vi "Manipulator Control.vi"() -> ()   [LabVIEW 2018]
uses:
  <vilib>/Platform/TimedLoop/XDataNode/timing_clust.ctl
  <vilib>/Platform/TimedLoop/XDataNode/nitl_modes.ctl
  <vilib>/Platform/TimedLoop/XDataNode/wakeup.ctl
  <vilib>/Analysis/baseanly.llb/Mean (DBL).vi
  <extravilib>/ChannelInstances/Tag-a[.](dbl)/Read With Abort.vi
  <extravilib>/ChannelInstances/Tag-bool/Read With Abort.vi
  <extravilib>/ChannelInstances/Tag-a[.](dbl)/Write With Abort.vi
  <extravilib>/ChannelInstances/Tag-bool/Write With Abort.vi
  <extravilib>/ChannelInstances/Tag-a[.](dbl)/Instantiate.vi
  <extravilib>/ChannelInstances/Tag-bool/Instantiate.vi
  <extravilib>/ChannelInstances/Tag-a[.](dbl)/EndpointRead.vi
  <extravilib>/ChannelInstances/Tag-bool/EndpointRead.vi
  <extravilib>/ChannelInstances/Tag-a[.](dbl)/Endpoint.vi
  <extravilib>/ChannelInstances/Tag-bool/Endpoint.vi
  <vilib>/Platform/TimedLoop/XDataNode/XDataNode.xnode
  <extravilib>/ChannelInstances/Tag-a[.](dbl).lvlib
  <extravilib>/ChannelInstances/Tag-bool.lvlib
  <vilib>/Platform/TimedLoop/XDataNode/XDNodeRunTimeDep.lvlib
  <vilib>/Analysis/NI_AALBase.lvlib
panel:
  in  "Derivative 1":dbl(slide)=6.0 min=0.0 max=10.0 step=0.1 scale=0.0..10.0
  in  "Integral 1":dbl(slide)=10.0 min=0.0 max=100.0 step=1.0 scale=0.0..100.0
  in  "Proportional 1":dbl(slide)=85.0 min=0.0 max=200.0 step=1.0 scale=0.0..200.0
  in  "Derivative 0":dbl(slide)=6.0 min=0.0 max=10.0 step=0.1 scale=0.0..10.0
  in  "Integral 0":dbl(slide)=10.0 min=0.0 max=100.0 step=1.0 scale=0.0..100.0
  out "Mean Task-Space \nerror (cm)":dbl=0.12500458479740745
  in  "Start Test":bool
  in  "Trajectory":enum16{"Circle", "Square"}(ring)
  in  "Stop Button":bool
  out "Calibrated":bool=TRUE
  out "Number of loops \ncompleted":i32=27
  in  "Error Threshold\n (cm)":dbl=0.3 format="%#_13g"
  in  "Proportional 0":dbl(slide)=85.0 min=0.0 max=200.0 step=1.0 scale=0.0..200.0
  out "Task-space Error":dbl(graph)=0.125479420396201
  out "Motor Voltage":T1(graph)={"element[0]"=-1.413534066833547, "element[1]"=1.33132478046187, "element[2]"=0.0, "element[3]"=0.0, "element[4]"=0.0, "element[5]"=0.0, "element[6]"=0.0, "element[7]"=0.0, "element[8]"=0.0}
  out "End-effector Trajectory":cluster{dbl[], dbl[]}[](graph)=[{[0.0, 0.0, 0.0, 0.0, 0.0, 0.0, 0.0, 0.0, 0.0, 0.0, 0.0, 0.0, 0.0, 0.0, 0.0, 0.0, 0.0, 0.0, 0.0, 0.0, 0.0, 0.0, 0.0, 0.0, 0.0, 0.0, 0.0, 0.0, 0.0, 0.0, 0.0, 0.0, 0.0, 0.0, 0.0, 0.0, 0.0, 0.0, 0.0, 0.0, 0.0, 0.0, 0.0, 0.0, 0.0, 0.0, 0.0, 0.0, 0.0, 0.0, 0.0, 0.0, 0.0, 0.0, 0.0, 0.0, 0.0, 0.0, 0.0, 0.0, 0.0, 0.0, 0.0, 0.0, 0.0, 0.0, 0.0, 0.0, 0.0, 0.0, 0.0, 0.0, 0.0, 0.0, 0.0, 0.0, 0.0, 0.0, 0.0, 0.0, 0.0, 0.0, 0.0, 0.0, 0.0, 0.0, 0.0, 0.0, 0.0, 0.0, 0.0, 0.0, 0.0, 0.0, 0.0, 0.0, 0.0, 0.0, 0.0, 0.0, 0.0, 0.0, 0.0, 0.0, 0.0, 0.0, 0.0, 0.0, 0.0, 0.0, 0.0, 0.0, 0.0, 0.0, 0.0, 0.0, 0.0, 0.0, 0.0, 0.0, 0.0, 0.0, 0.0, 0.0, 0.0, 0.0, 0.0, 0.0], [10.0, 10.0, 10.0, 10.0, 10.0, 10.0, 10.0, 10.0, 10.0, 10.0, 10.0, 10.0, 10.0, 10.0, 10.0, 10.0, 10.0, 10.0, 10.0, 10.0, 10.0, 10.0, 10.0, 10.0, 10.0, 10.0, 10.0, 10.0, 10.0, 10.0, 10.0, 10.0, 10.0, 10.0, 10.0, 10.0, 10.0, 10.0, 10.0, 10.0, 10.0, 10.0, 10.0, 10.0, 10.0, 10.0, 10.0, 10.0, 10.0, 10.0, 10.0, 10.0, 10.0, 10.0, 10.0, 10.0, 10.0, 10.0, 10.0, 10.0, 10.0, 10.0, 10.0, 10.0, 10.0, 10.0, 10.0, 10.0, 10.0, 10.0, 10.0, 10.0, 10.0, 10.0, 10.0, 10.0, 10.0, 10.0, 10.0, 10.0, 10.0, 10.0, 10.0, 10.0, 10.0, 10.0, 10.0, 10.0, 10.0, 10.0, 10.0, 10.0, 10.0, 10.0, 10.0, 10.0, 10.0, 10.0, 10.0, 10.0, 10.0, 10.0, 10.0, 10.0, 10.0, 10.0, 10.0, 10.0, 10.0, 10.0, 10.0, 10.0, 10.0, 10.0, 10.0, 10.0, 10.0, 10.0, 10.0, 10.0, 10.0, 10.0, 10.0, 10.0, 10.0, 10.0, 10.0, 10.0]}, {[0.10886586911216156, 0.10886586911216156, 0.10886586911216156, 0.10886586911216156, 0.10886586911216156, 0.10338675897126315, 0.10338675897126315, 0.10886586911216156, 0.10886586911216156, 0.10886586911216156, 0.10886586911216156, 0.10886586911216156, 0.10886586911216156, 0.10338675897126315, 0.10338675897126315, 0.12367237442525791, 0.10886586911216156, 0.10886586911216156, 0.10886586911216156, 0.10886586911216156, 0.10886586911216156, 0.10338675897126315, 0.10338675897126315, 0.10338675897126315, 0.10338675897126315, 0.10338675897126315, 0.10886586911216156, 0.12914220502365836, 0.10886586911216156, 0.10886586911216156, 0.10886586911216156, 0.10886586911216156, 0.10338675897126315, 0.10338675897126315, 0.10338675897126315, 0.12914220502365836, 0.10886586911216156, 0.12914220502365836, 0.12914220502365836, 0.10338675897126315, 0.12367237442525791, 0.12367237442525791, 0.10886586911216156, 0.10886586911216156, 0.10886586911216156, 0.10886586911216156, 0.12914220502365836, 0.12914220502365836, 0.10886586911216156, 0.10886586911216156, 0.10886586911216156, 0.10886586911216156, 0.12367237442525791, 0.12367237442525791, 0.10338675897126315, 0.12914220502365836, 0.10886586911216156, 0.12914220502365836, 0.12914220502365836, 0.10886586911216156, 0.12914220502365836, 0.12914220502365836, 0.10886586911216156, 0.10886586911216156, 0.10338675897126315, 0.10886586911216156, 0.12914220502365836, 0.12914220502365836, 0.12914220502365836, 0.12914220502365836, 0.12914220502365836, 0.10886586911216156, 0.12914220502365836, 0.12367237442525791, 0.10886586911216156, 0.12367237442525791, 0.10886586911216156, 0.12914220502365836, 0.12914220502365836, 0.12914220502365836, 0.12914220502365836, 0.10886586911216156, 0.12914220502365836, 0.12914220502365836, 0.12367237442525791, 0.10886586911216156, 0.10338675897126315, 0.12914220502365836, 0.12914220502365836, 0.12914220502365836, 0.12914220502365836, 0.12914220502365836, 0.12914220502365836, 0.10886586911216156, 0.12914220502365836, 0.10886586911216156, 0.12367237442525791, 0.12367237442525791, 0.12914220502365836, 0.12367237442525791, 0.12914220502365836, 0.12914220502365836, 0.12914220502365836, 0.12914220502365836, 0.12914220502365836, 0.12914220502365836, 0.12914220502365836, 0.12914220502365836, 0.12914220502365836, 0.12367237442525791, 0.12914220502365836, 0.12914220502365836, 0.12914220502365836, 0.12914220502365836, 0.12914220502365836, 0.12914220502365836, 0.12914220502365836, 0.12914220502365836, 0.12914220502365836, 0.12914220502365836, 0.12914220502365836, 0.12914220502365836, 0.12914220502365836, 0.12914220502365836, 0.12914220502365836, 0.12914220502365836, 0.12914220502365836, 0.12914220502365836], [9.93760362602346, 9.93760362602346, 9.93760362602346, 9.93760362602346, 9.93760362602346, 9.91519089242297, 9.91519089242297, 9.93760362602346, 9.93760362602346, 9.93760362602346, 9.93760362602346, 9.93760362602346, 9.93760362602346, 9.91519089242297, 9.91519089242297, 9.896688321217006, 9.93760362602346, 9.93760362602346, 9.93760362602346, 9.93760362602346, 9.93760362602346, 9.91519089242297, 9.91519089242297, 9.91519089242297, 9.91519089242297, 9.91519089242297, 9.93760362602346, 9.919095342569769, 9.93760362602346, 9.93760362602346, 9.93760362602346, 9.93760362602346, 9.91519089242297, 9.91519089242297, 9.91519089242297, 9.919095342569769, 9.93760362602346, 9.919095342569769, 9.919095342569769, 9.91519089242297, 9.896688321217006, 9.896688321217006, 9.93760362602346, 9.93760362602346, 9.93760362602346, 9.93760362602346, 9.919095342569769, 9.919095342569769, 9.93760362602346, 9.93760362602346, 9.93760362602346, 9.93760362602346, 9.896688321217006, 9.896688321217006, 9.91519089242297, 9.919095342569769, 9.93760362602346, 9.919095342569769, 9.919095342569769, 9.93760362602346, 9.919095342569769, 9.919095342569769, 9.93760362602346, 9.93760362602346, 9.91519089242297, 9.93760362602346, 9.919095342569769, 9.919095342569769, 9.919095342569769, 9.919095342569769, 9.919095342569769, 9.93760362602346, 9.919095342569769, 9.896688321217006, 9.93760362602346, 9.896688321217006, 9.93760362602346, 9.919095342569769, 9.919095342569769, 9.919095342569769, 9.919095342569769, 9.93760362602346, 9.919095342569769, 9.919095342569769, 9.896688321217006, 9.93760362602346, 9.91519089242297, 9.919095342569769, 9.919095342569769, 9.919095342569769, 9.919095342569769, 9.919095342569769, 9.919095342569769, 9.93760362602346, 9.919095342569769, 9.93760362602346, 9.896688321217006, 9.896688321217006, 9.919095342569769, 9.896688321217006, 9.919095342569769, 9.919095342569769, 9.919095342569769, 9.919095342569769, 9.919095342569769, 9.919095342569769, 9.919095342569769, 9.919095342569769, 9.919095342569769, 9.896688321217006, 9.919095342569769, 9.919095342569769, 9.919095342569769, 9.919095342569769, 9.919095342569769, 9.919095342569769, 9.919095342569769, 9.919095342569769, 9.919095342569769, 9.919095342569769, 9.919095342569769, 9.919095342569769, 9.919095342569769, 9.919095342569769, 9.919095342569769, 9.919095342569769, 9.919095342569769, 9.919095342569769]}]
  # "Mechatronic Systems Board"
  # "Manipulator Control"
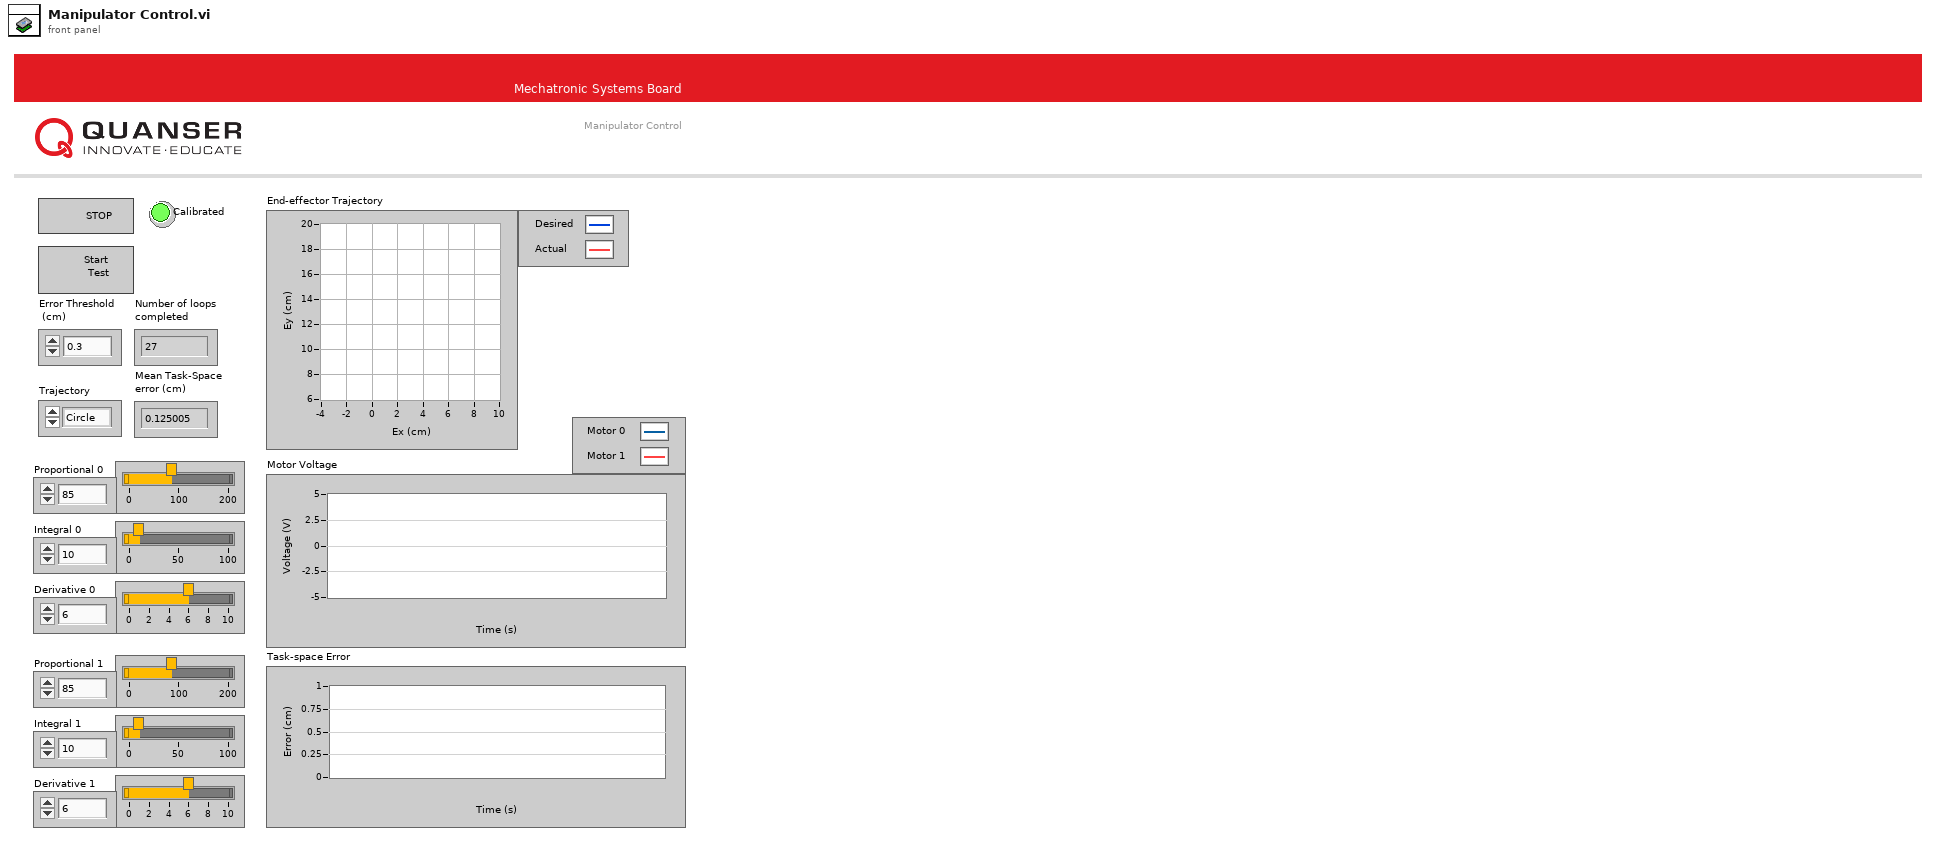
[diagram p1: front panel]
types:
  T1 = cluster{"element[0]":dbl, "element[1]":dbl, "element[2]":dbl, "element[3]":dbl, "element[4]":dbl, "element[5]":dbl, "element[6]":dbl, "element[7]":dbl, "element[8]":dbl}
  T2 = enum16{"Initialize", "Ready", "Start", "Move", "Wait", "Done"}
  T3 = typedef "QNET MS IO Cluster.ctl" = cluster{"Error":errorcluster, "Encoder Calibration Values":i32[], "Update Calibration":bool, "JPEG Resolutions":u16, "Raw Resolutions":u16, "Image Mode":enum16{"RAW RGB", "RAW Gray Scale", "JPEG"}, "FPGA Ref":refnum<k20>}
  T4 = typedef "XDNodeRunTimeDep.lvlib/timing_clust.ctl" = cluster{"Expected End [f-1]":u64, "Actual End [f-1]":u64, "Finished Late? [f-1]":bool, "Expected End [i-1]":u64, "Actual End [i-1]":u64, "Finished Late? [i-1]":bool, "Expected Start [i]":u64, "Actual Start [i]":u64, "Expected Start [f]":u64, "Actual Start [f]":u64, "Source Name":string, "Structure Name":string, "Period":i64, "Deadline":i64, "Offset":i64, "Start":i64, "Priority":i32, "Timeout":i32, "Mode":T5, "Wakeup Reason":T6, "Error":errorcluster, "Source Type":string, "Secondary Source Type":string, "Global End Time":u64, "Global Start Time":u64, "Frame Duration":u64, "Iteration Duration":u64, "Assigned CPU":i32, "I/O Scan Engine Mode":u32}
  T5 = typedef "XDNodeRunTimeDep.lvlib/nitl_modes.ctl" = enum32{"No Change", "Process missed periods, maintain original phase", "Discard missed periods, maintain original phase", "Process missed periods, ignore original phase", "Discard missed periods, ignore original phase"}
  T6 = typedef "XDNodeRunTimeDep.lvlib/wakeup.ctl" = enum32{"Normal", "Aborted", "Asynchronous wakeup", "Timing source error", "Timed loop error", "Timeout"}
  T7 = enum8{"Enabled", "Disabled", "Disabled and Grayed Out"}
  T8 = typedef "Tag-bool.lvlib/))Channel.ctl" = refnum<queue>
  T9 = typedef "Tag-a[.](dbl).lvlib/))Channel.ctl" = refnum<queue>
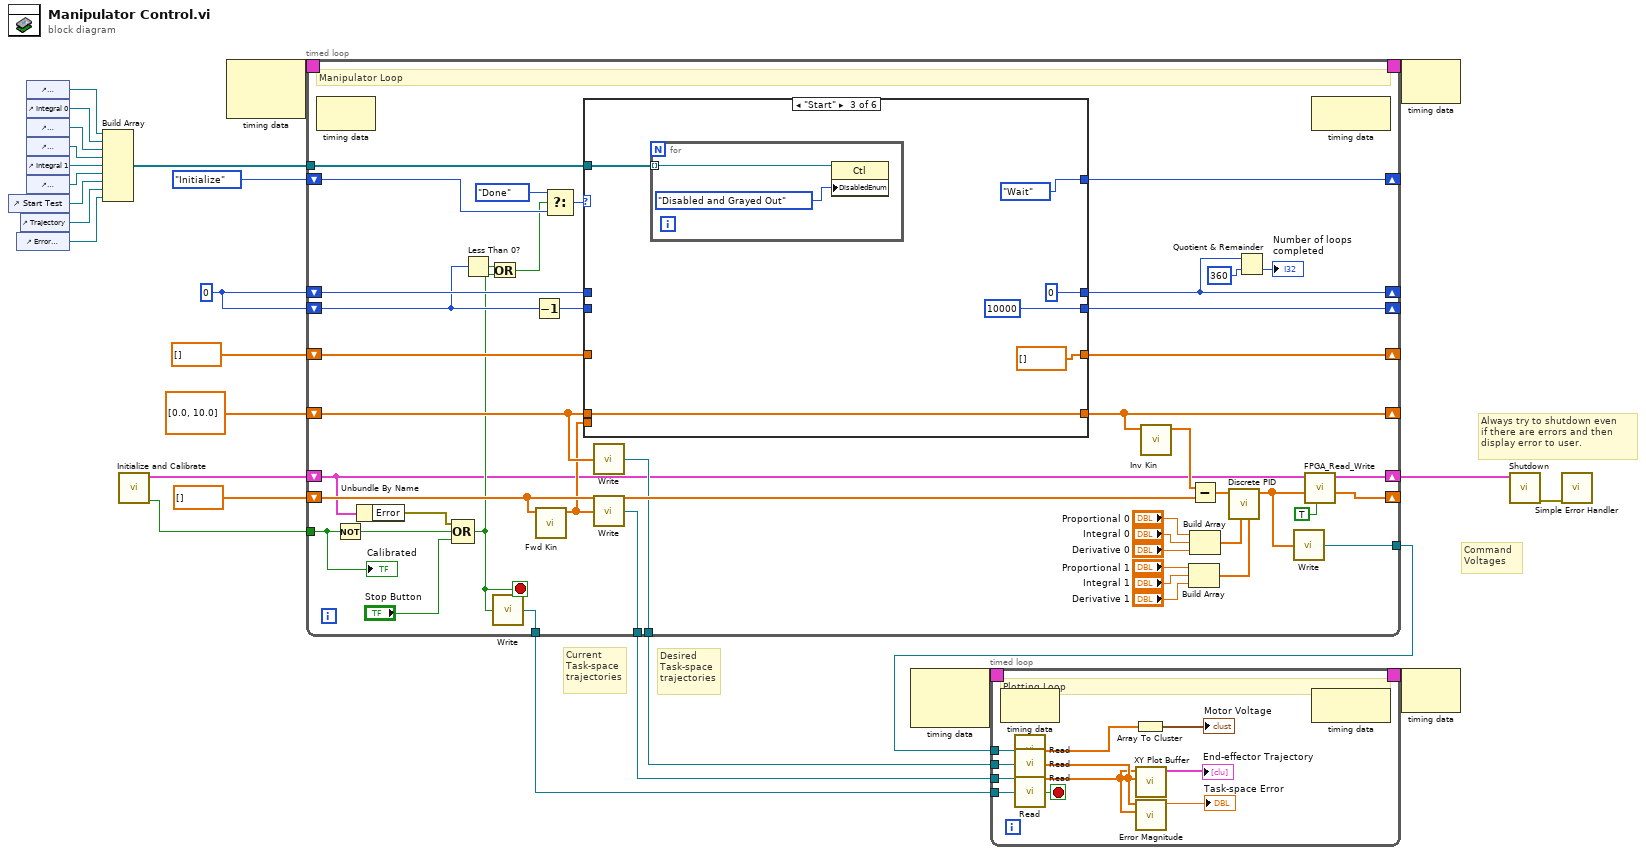
[diagram p0: block diagram]
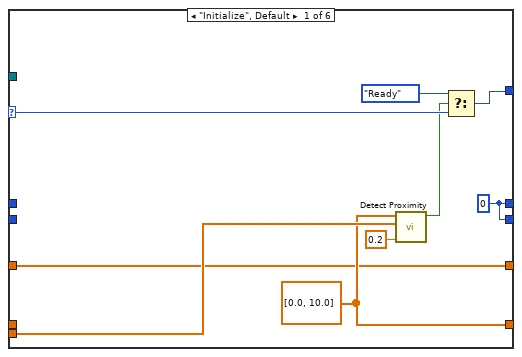
[diagram p2: hidden frame]
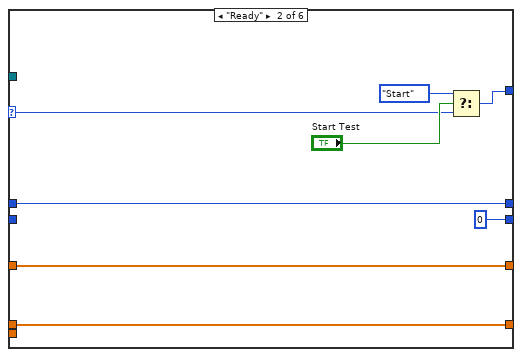
[diagram p3: hidden frame]
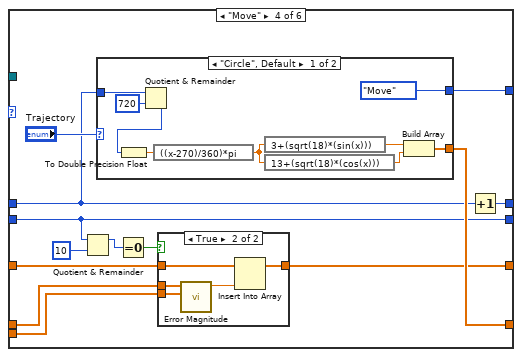
[diagram p4: hidden frame]
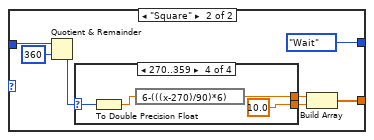
[diagram p6: hidden frame]
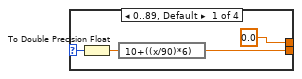
[diagram p7: hidden frame]
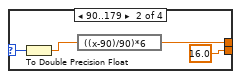
[diagram p8: hidden frame]
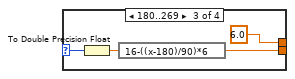
[diagram p9: hidden frame]
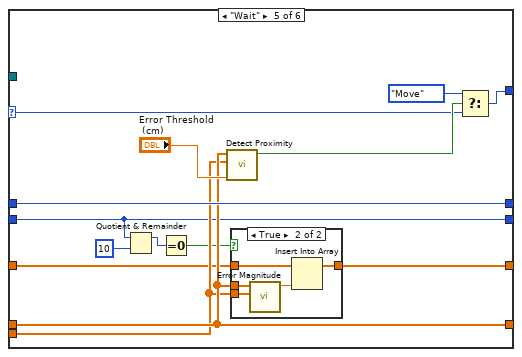
[diagram p10: hidden frame]
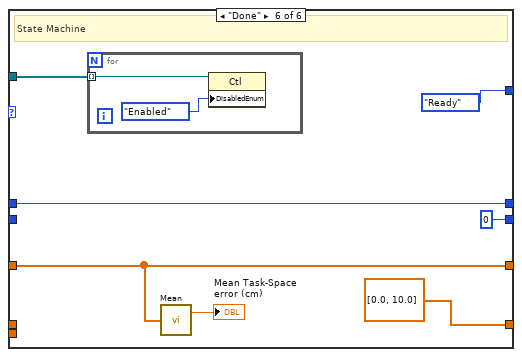
[diagram p12: hidden frame]
diagram:
  w9 = 0
  # "Command\nVoltages"
  # "Current\nTask-space\ntrajectories"
  # "Desired\nTask-space\ntrajectories"
  # "Always try to shutdown even \nif there are errors and then \ndisplay error to user."
  n1 = control-ref of="Start Test"() -> (w14:refnum<vi>)
  n2 = control-ref of="Error Threshold\n (cm)"() -> (w12:refnum<vi>)
  n3 = control-ref of="Trajectory"() -> (w13:refnum<vi>)
  n4 = control-ref of="Proportional 0"() -> (w15:refnum<vi>)
  n5 = control-ref of="Integral 0"() -> (w7:refnum<vi>)
  n6 = control-ref of="Derivative 0"() -> (w6:refnum<vi>)
  n7 = control-ref of="Proportional 1"() -> (w5:refnum<vi>)
  n8 = control-ref of="Integral 1"() -> (w4:refnum<vi>)
  n9 = control-ref of="Derivative 1"() -> (w3:refnum<vi>)
  n10 = Build Array(w15, w7, w6, w5, w4, w3, w14, w13, w12) -> (w11:refnum<vi>[])
  n11 = call "Initialize and Calibrate.vi"() -> ("Calibrated"=w19:bool, "IO Cluster"=w24:T3)  [unwired: 10 in]
  n12 = node-c288() -> (w26:T4)  [unwired: 2 in]
  n13 = timed-loop {
    timing: w26 -> [_]
    timing-out: [_] -> w25
    shift-right: [w66] -> w23
    shift-left: w24 -> [w29]
    shift-right: [w63] -> _
    shift-left: dbl[] [] ("Joint Coordinates (rad)") -> [w61]
    shift-right: [w64] -> _
    shift-left: T2."Initialize" -> [w47]
    shift-right: [w62] -> _
    shift-left: dbl[] [0.0, 10.0] -> [w60]
    shift-right: [w52] -> _
    shift-left: w9 -> [w65]
    tunnel: w19 -> [w32]
    tunnel: [w59] -> w18
    tunnel: [w58] -> w17
    tunnel: [w57] -> w16
    tunnel: w11 -> [w54]
    shift-right: [w48] -> _
    shift-left: dbl[] [] ("Joint Coordinates (rad)") -> [w49]
    shift-right: [w46] -> _
    shift-left: w9 -> [w43]
    tunnel: [w40] -> w8
    stop <- w30 stop-if-true
    # "Manipulator Loop"
    n14 = node-c288() -> ()  [unwired: 1 in, 1 out]
    n15 = Not(x=w32) -> (.not. x?=w31:bool)
    n16 = Unbundle By Name(w29) -> ("Error"=w28:errorcluster)
    n17 = Compound Arithmetic op=OR(w28, w31, "Stop Button") -> (w30:bool)
    n18 = Less Than 0?(x=w43) -> (x < 0?=w44:bool)
    n19 = Or(x=w44, y=w30) -> (x .or. y?=w42:bool)
    n20 = call <extravilib>:"Write.vi"("element"=w30) -> ("channel"=w57:T8)  [unwired: 1 out]
    n21 = Decrement(x=w43) -> (x-1=w45:i32)
    n22 = call "Fwd Kin.vi"("Joint Coordinates (rad)"=w61) -> ("Task Coordinates (cm)"=w53:dbl[])  [unwired: 9 in, 1 out]
    n23 = Select(t=T2."Done", s=w42, f=w47) -> (s? t:f=w56:T2)
    n24 = case shown="\"Start\"" w56 {
      selector: w56 -> [w79 w85 _ _ w158 _]
      tunnel: w65 -> [_ w81 _ w97 w161 w174]
      tunnel: [w72 w81 0 w109 w161 w174] -> w52
      tunnel: [w76 w88 w94 w108 w155 dbl[] [0.0, 10.0]] -> w62
      tunnel: w60 -> [_ w88 w94 w106 w155 _]
      tunnel: w53 -> [w80 _ _ w105 w154 _]
      tunnel: [w78 w84 T2."Wait" w98 w157 T2."Ready" ("t")] -> w64
      tunnel: w54 -> [_ _ w91 _ _ w173]
      tunnel: w49 -> [w73 w83 _ w104 w153 w170]
      tunnel: w45 -> [_ _ _ w102 w149 _]
      tunnel: [w72 0 10000 w102 w149 0] -> w46
      tunnel: [w73 w83 dbl[] [] ("Joint Coordinates (rad)") w103 w152 w170] -> w48
      frame "Initialize", Default {
        w72 = 0
        w76 = dbl[] [0.0, 10.0]
        n25 = call "Detect Proximity.vi"("Threshold"=0.2, "E current"=w80, "E desired"=w76) -> ("Close Enough?"=w77:bool)  [unwired: 8 in]
        n26 = Select(t=T2."Ready", s=w77, f=w79) -> (s? t:f=w78:T2)
      }
      frame "Ready" {
        n27 = Select(t=T2."Start", s="Start Test", f=w85) -> (s? t:f=w84:T2)
      }
      frame "Start" {
        n28 = for {
          tunnel: w91 -> [w96] mode=indexing
          n29 = property class="Ctl"(reference=w96, "DisabledEnum"=T7."Disabled and Grayed Out" ("Disabled")) -> ()  [unwired: 1 in, 2 out]
        }
      }
      frame "Move" {
        n30 = Quotient & Remainder(x=w102, y=10) -> (x-y*floor(x/y)=w100:i32)  [unwired: 1 out]
        n31 = case shown="\"Circle\", Default" "Trajectory" {
          tunnel: [w124 w129] -> w108
          tunnel: [T2."Move" T2."Wait"] -> w98
          tunnel: w97 -> [w117 w126]
          frame "Circle", Default {
            n32 = Quotient & Remainder(x=w117, y=720) -> (x-y*floor(x/y)=w116:i32)  [unwired: 1 out]
            n33 = To Double Precision Float(number=w116) -> (double precision float=w123:dbl)
            n34 = expression code="((x-270)/360)*pi" ("degrees to radians")(w123) -> (w122:dbl)
            n35 = expression code="3+(sqrt(18)*(sin(x)))"(w122) -> (w121:dbl)
            n36 = expression code="13+(sqrt(18)*(cos(x)))"(w122) -> (w120:dbl)
            n37 = Build Array(w121, w120) -> (w124:dbl[])
          }
          frame "Square" {
            n38 = Quotient & Remainder(x=w126, y=360) -> (x-y*floor(x/y)=w125:i32)  [unwired: 1 out]
            n39 = case shown="270..359" w125 {
              selector: w125 -> [w134 w138 w140 w146]
              tunnel: [0.0 w136 6.0 w145] -> w131
              tunnel: [w132 16.0 w142 10.0] -> w130
              frame 0..89, Default {
                n40 = To Double Precision Float(number=w134) -> (double precision float=w133:dbl)
                n41 = expression code="10+((x/90)*6)"(w133) -> (w132:dbl)
              }
              frame 90..179 {
                n42 = To Double Precision Float(number=w138) -> (double precision float=w137:dbl)
                n43 = expression code="((x-90)/90)*6"(w137) -> (w136:dbl)
              }
              frame 180..269 {
                n44 = To Double Precision Float(number=w140) -> (double precision float=w141:dbl)
                n45 = expression code="16-((x-180)/90)*6"(w141) -> (w142:dbl)
              }
              frame 270..359 {
                n46 = To Double Precision Float(number=w146) -> (double precision float=w144:dbl)
                n47 = expression code="6-(((x-270)/90)*6)"(w144) -> (w145:dbl)
              }
            }
            n48 = Build Array(w131, w130) -> (w129:dbl[])
          }
        }
        n49 = Equal To 0?(x=w100) -> (x = 0?=w99:bool)
        n50 = case shown="True" w99 {
          tunnel: w106 -> [_ w115]
          tunnel: w105 -> [_ w114]
          tunnel: w104 -> [w110 w112]
          tunnel: [w110 w111] -> w103
          frame False {
          }
          frame True {
            n51 = call "Error Magnitude.vi"("Actual Task Coordinates (cm)"=w114, "Desired Task Coordinates (cm)"=w115) -> ("Task-space\nError"=w113:dbl)  [unwired: 9 in]
            n52 = Insert Into Array(array=w112, new element=w113) -> (w111:dbl[])  [unwired: 1 in]
          }
        }
        n53 = Increment(x=w97) -> (x+1=w109:i32)
      }
      frame "Wait" {
        n54 = Quotient & Remainder(x=w149, y=10) -> (x-y*floor(x/y)=w150:i32)  [unwired: 1 out]
        n55 = Equal To 0?(x=w150) -> (x = 0?=w148:bool)
        n56 = call "Detect Proximity.vi"("Threshold"="Error Threshold\n (cm)", "E current"=w154, "E desired"=w155) -> ("Close Enough?"=w159:bool)  [unwired: 8 in]
        n57 = case shown="True" w148 {
          tunnel: w155 -> [_ w167]
          tunnel: w154 -> [_ w166]
          tunnel: w153 -> [w162 w165]
          tunnel: [w162 w164] -> w152
          frame False {
          }
          frame True {
            n58 = call "Error Magnitude.vi"("Actual Task Coordinates (cm)"=w166, "Desired Task Coordinates (cm)"=w167) -> ("Task-space\nError"=w163:dbl)  [unwired: 9 in]
            n59 = Insert Into Array(array=w165, new element=w163) -> (w164:dbl[])  [unwired: 1 in]
          }
        }
        n60 = Select(t=T2."Move", s=w159, f=w158) -> (s? t:f=w157:T2)
      }
      frame "Done" {
        # "State Machine"
        n61 = for {
          tunnel: w173 -> [w176] mode=indexing
          n62 = property class="Ctl"(reference=w176, "DisabledEnum"=T7."Enabled" ("Disabled")) -> ()  [unwired: 1 in, 2 out]
        }
        n63 = call-poly <vilib>:"Mean.vi"("X"=w170) -> ("mean"=→"Mean Task-Space \nerror (cm)":dbl)  [unwired: 1 out]
      }
    }
    n64 = call <extravilib>:"Write.vi"("element"=w60) -> ("channel"=w58:T9)  [unwired: 1 out]
    n65 = call <extravilib>:"Write.vi"("element"=w53) -> ("channel"=w59:T9)  [unwired: 1 out]
    n66 = call "Inv Kin.vi"("Task Coordinates (cm)"=w62) -> ("Joint Coordinates (rad)"=w67:dbl[])  [unwired: 10 in]
    n67 = Build Array("Proportional 1", "Integral 1", "Derivative 1") -> (w34:dbl[])
    n68 = Subtract(x=w67, y=w61) -> (x-y=w69:dbl[])
    n69 = Build Array("Proportional 0", "Integral 0", "Derivative 0") -> (w70:dbl[])
    n70 = call "Discrete PID.vi"("Gains Motor 1"=w34, "Gains Motor 0"=w70, "Error Array"=w69) -> ("Voltage"=w41:dbl[])  [unwired: 8 in]
    n71 = Quotient & Remainder(x=w52, y=360) -> (floor(x/y)=→"Number of loops \ncompleted":i32)  [unwired: 1 out]
    n72 = call <extravilib>:"Write.vi"("element"=w41) -> ("channel"=w40:T9)  [unwired: 1 out]
    n73 = call "FPGA_Read_Write.vi"("Motors enabled?"=TRUE, "Commands"=w41, "IO Cluster In"=w29) -> ("Joint Coordinates (rad)"=w63:dbl[], "IO Cluster Out"=w66:T3)  [unwired: 5 in, 2 out]
    n74 = node-c288() -> ()  [unwired: 1 in, 1 out]
    "Calibrated" <- w32
  }
  n75 = node-c288() -> (w2:T4)  [unwired: 2 in]
  n76 = timed-loop {
    tunnel: w16 -> [w189]
    tunnel: w17 -> [w188]
    tunnel: w18 -> [w187]
    tunnel: w8 -> [w181]
    timing: w2 -> [_]
    timing-out: [_] -> w1
    stop <- w183 stop-if-true
    # "Plotting Loop"
    n77 = node-c288() -> ()  [unwired: 1 in, 1 out]
    n78 = call <extravilib>:"Read.vi"("channel"=w181) -> ("element"=w180:dbl[])  [unwired: 1 in, 1 out]
    n79 = call <extravilib>:"Read.vi"("channel"=w188) -> ("element"=w185:dbl[])  [unwired: 1 in, 1 out]
    n80 = call <extravilib>:"Read.vi"("channel"=w187) -> ("element"=w184:dbl[])  [unwired: 1 in, 1 out]
    n81 = call <extravilib>:"Read.vi"("channel"=w189) -> ("element"=w183:bool)  [unwired: 1 in, 1 out]
    n82 = Array To Cluster(array=w180) -> (cluster=→"Motor Voltage":T1)
    n83 = call "XY Plot Buffer.vi"("Desired"=w185, "Actual"=w184) -> ("Buffered Task Coordinates"=→"End-effector Trajectory":cluster{dbl[], dbl[]}[])  [unwired: 9 in]
    n84 = call "Error Magnitude.vi"("Actual Task Coordinates (cm)"=w184, "Desired Task Coordinates (cm)"=w185) -> ("Task-space\nError"=→"Task-space Error":dbl)  [unwired: 9 in]
    n85 = node-c288() -> ()  [unwired: 1 in, 1 out]
  }
  n86 = node-c288(w25) -> ()  [unwired: 1 out]
  n87 = node-c288(w1) -> ()  [unwired: 1 out]
  n88 = call "Shutdown.vi"("IO Cluster In"=w23) -> ("Error"=w27:errorcluster)  [unwired: 10 in]
  n89 = call <vilib>:"Simple Error Handler.vi"("error in (no error)"=w27) -> ()  [unwired: 4 in, 5 out]
